vi "myRIO__TCP_constants_byteRange_messageType_block.vi"() -> (2 "output_Block_byte":u8=66, 3 "output_Block_char":string="B")   [LabVIEW 2014]
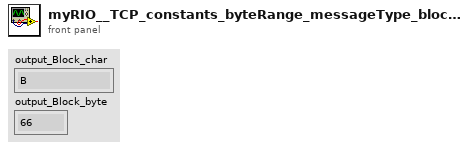
[diagram p1: front panel]
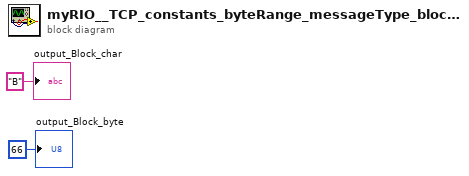
[diagram p0: block diagram]
diagram:
  "output_Block_char" <- "B"
  "output_Block_byte" <- u8 66
